vi "rs3 send_and_receive_raw_data3.vi"(0 "device in":u64=2630156989648, 2 "x1,y1,x2,y2":sgl[](array[numeric])=[0.0, 0.0, 0.0, 0.0], 5 "Send command":T3(ring)=enum."Distortion Centers", 7 "Input data":u32 format="%x", 9 "Input Intermediate Calibration Parameters":T2={"fx"=0.4987139, "fy"=0.7959354, "px"=0.49842373, "py"=0.49641025, "k left"=[-0.056493655, 0.06423295, 0.00075629074, -0.00050474313, -0.019832378], "fx2"=0.50020504, "fy2"=0.7982992, "py2"=0.5080532, "px2"=0.4993604, "k right"=[-0.056605, 0.065333016, 0.00090795365, 4.2479092e-05, -0.020946281], "RLeft"=[0.9999964, 0.001770121, -0.002005104, -0.0017697959, 0.9999984, 0.0001639397, 0.0020053908, -0.00016039048, 0.999998], "Rright"=[0.999991, -0.0020914313, -0.0036981972, 0.0020908315, 0.9999978, -0.00016603176, 0.0036985364, 0.00015829796, 0.99999315], "baseline"=-49.819336, "useBrownModel"=1, "1280x720"=[641.0225, 641.0225, 634.87134, 362.7353]}, 11 "error in (no error)":errorcluster, 13 "Calibration table input":T1={"version"=3, "table type"=60479, "table size"=496, "full version"=67109888, "crc32"=3963612841, "baseline"=-54.831806, "model"=1, "fx left"=917.7658, "fy left"=915.4345, "px left"=631.39185, "py left"=376.6227, "py right"=364.3492, "px right"=651.2822, "fy right"=921.49005, "fx right"=923.5849, "k left"=[0.13533829, -0.40519878, 0.0008784002, -0.0011180333, 0.3588802], "k right"=[0.12740475, -0.39763576, 0.00037952562, -0.0022863527, 0.35284942], "RLeft"=[0.9999986, 0.0009555143, -0.001359244, -0.0009574645, 0.9999985, -0.001434832, 0.001357871, 0.0014361315, 0.99999803], "Rright"=[0.99998456, -0.0019937593, -0.0051888847, 0.002001206, 0.99999696, 0.0014302958, 0.0051860176, -0.0014406577, 0.9999855], "uint8 reserved1"=[0, 0, 0, 0, 0, 0, 0, 0, 0, 0, 0, 0, 0, 0, 0, 0, 0, 0, 0, 0, 0, 0, 0, 0, 0, 0, 0, 0, 0, 0, 0, 0, 0, 0, 0, 0, 0, 0, 0, 0, 0, 0, 0, 0, 0, 0, 0, 0, 0, 0, 0, 0, 0, 0, 0, 0, 0, 0, 0, 0, 0, 0, 0, 0, 0, 0, 0, 0, 0, 0, 0, 0, 0, 0, 0, 0, 0, 0, 0, 0, 0, 0, 0, 0, 0, 0, 0, 0], "uint8 reserved2"=[0, 0, 0, 0, 0, 0, 0, 0, 0, 0, 0, 0, 0, 0, 0, 0, 0, 0, 0, 0, 0, 0, 0, 0, 0, 0, 0, 0, 0, 0, 0, 0, 0, 0, 0, 0, 0, 0, 0, 0, 0, 0, 0, 0, 0, 0, 0, 0, 0, 0, 0, 0, 0, 0, 0, 0, 0, 0, 0, 0, 0, 0, 0, 0], "1920x1080"=[1428.9095, 1428.9095, 951.85925, 556.0496], "1280x720"=[952.6064, 952.6064, 634.5728, 370.69974], "640x480"=[635.0709, 635.0709, 316.38187, 247.13316], "848x480"=[635.0709, 635.0709, 420.38187, 247.13316], "640x360"=[476.3032, 476.3032, 317.2864, 185.34987], "424x240"=[317.53546, 317.53546, 210.19093, 123.56658], "320x240"=[317.53546, 317.53546, 158.19093, 123.56658], "480x270"=[357.2274, 357.2274, 237.96481, 139.0124], "1280x800"=[1058.4515, 1058.4515, 633.9698, 411.8886], "960x540"=[714.4548, 714.4548, 475.92963, 278.0248], "Reserved1"=[714.4548, 714.4548, 475.92963, 278.0248], "Reserved 2"=[714.4548, 714.4548, 475.92963, 278.0248]} {"crc32" format="%x"}, 14 "Custom array":u8[](array[numeric])=[20, 1, 0, 0, 81, 0, 0, 0, 0, 0, 0, 0, 0, 0, 0, 0, 0, 0, 0, 0, 0, 0, 0, 0, 110, 87, 255, 62, 108, 194, 75, 63, 101, 49, 255, 62, 124, 41, 254, 62, 228, 101, 103, 189, 145, 140, 131, 61, 208, 65, 70, 58, 189, 80, 4, 186, 131, 119, 162, 188, 112, 13, 0, 63, 86, 93, 76, 63, 43, 172, 255, 62, 198, 15, 2, 63, 165, 218, 103, 189, 81, 205, 133, 61, 189, 3, 110, 58, 148, 43, 50, 56, 137, 151, 171, 188, 196, 255, 127, 63, 104, 3, 232, 58, 16, 104, 3, 187, 127, 248, 231, 186, 229, 255, 127, 63, 58, 231, 43, 57, 224, 108, 3, 59, 126, 46, 40, 185, 222, 255, 127, 63, 105, 255, 127, 63, 101, 16, 9, 187, 116, 93, 114, 187, 85, 6, 9, 59, 219, 255, 127, 63, 208, 24, 46, 185, 37, 99, 114, 59, 201, 252, 37, 57, 141, 255, 127, 63, 0, 71, 71, 194, 1, 0, 0, 0, 0, 0, 0, 0, 0, 0, 0, 0, 0, 0, 0, 0, 0, 0, 0, 0, 0, 0, 0, 0, 0, 0, 0, 0, 0, 0, 0, 0, 0, 0, 0, 0, 0, 0, 0, 0, 0, 0, 0, 0, 0, 0, 0, 0, 0, 0, 0, 0, 0, 0, 0, 0, 0, 0, 0, 0, 0, 0, 0, 0, 0, 0, 0, 0, 0, 0, 0, 0, 0, 0, 0, 0, 0, 0, 0, 0, 0, 0, 0, 0, 0, 0, 0, 0, 0, 0, 0, 0, 113, 65, 32, 68, 113, 65, 32, 68, 196, 183, 30, 68, 30, 94, 181, 67] format="%x") -> (1 "size(s)":i32=280, 3 "Output Calibration table":T1={"version"=3, "table type"=60479, "table size"=496, "full version"=67109888, "crc32"=3963612841, "baseline"=-54.831806, "model"=1, "fx left"=917.7658, "fy left"=915.4345, "px left"=631.39185, "py left"=376.6227, "py right"=364.3492, "px right"=651.2822, "fy right"=921.49005, "fx right"=923.5849, "k left"=[0.13533829, -0.40519878, 0.0008784002, -0.0011180333, 0.3588802], "k right"=[0.12740475, -0.39763576, 0.00037952562, -0.0022863527, 0.35284942], "RLeft"=[0.9999986, 0.0009555143, -0.001359244, -0.0009574645, 0.9999985, -0.001434832, 0.001357871, 0.0014361315, 0.99999803], "Rright"=[0.99998456, -0.0019937593, -0.0051888847, 0.002001206, 0.99999696, 0.0014302958, 0.0051860176, -0.0014406577, 0.9999855], "uint8 reserved1"=[0, 0, 0, 0, 0, 0, 0, 0, 0, 0, 0, 0, 0, 0, 0, 0, 0, 0, 0, 0, 0, 0, 0, 0, 0, 0, 0, 0, 0, 0, 0, 0, 0, 0, 0, 0, 0, 0, 0, 0, 0, 0, 0, 0, 0, 0, 0, 0, 0, 0, 0, 0, 0, 0, 0, 0, 0, 0, 0, 0, 0, 0, 0, 0, 0, 0, 0, 0, 0, 0, 0, 0, 0, 0, 0, 0, 0, 0, 0, 0, 0, 0, 0, 0, 0, 0, 0, 0], "uint8 reserved2"=[0, 0, 0, 0, 0, 0, 0, 0, 0, 0, 0, 0, 0, 0, 0, 0, 0, 0, 0, 0, 0, 0, 0, 0, 0, 0, 0, 0, 0, 0, 0, 0, 0, 0, 0, 0, 0, 0, 0, 0, 0, 0, 0, 0, 0, 0, 0, 0, 0, 0, 0, 0, 0, 0, 0, 0, 0, 0, 0, 0, 0, 0, 0, 0], "1920x1080"=[1428.9095, 1428.9095, 951.85925, 556.0496], "1280x720"=[952.6064, 952.6064, 634.5728, 370.69974], "640x480"=[635.0709, 635.0709, 316.38187, 247.13316], "848x480"=[635.0709, 635.0709, 420.38187, 247.13316], "640x360"=[476.3032, 476.3032, 317.2864, 185.34987], "424x240"=[317.53546, 317.53546, 210.19093, 123.56658], "320x240"=[317.53546, 317.53546, 158.19093, 123.56658], "480x270"=[357.2274, 357.2274, 237.96481, 139.0124], "1280x800"=[1058.4515, 1058.4515, 633.9698, 411.8886], "960x540"=[714.4548, 714.4548, 475.92963, 278.0248], "Reserved1"=[714.4548, 714.4548, 475.92963, 278.0248], "Reserved 2"=[714.4548, 714.4548, 475.92963, 278.0248]} {"crc32" format="%x"}, 4 "Sent Command":u8[](array[numeric])=[20, 0, 171, 205, 21, 0, 0, 0, 25, 0, 0, 0, 0, 0, 0, 0, 0, 0, 0, 0, 0, 0, 0, 0] format="%x", 6 "Response array":u8[](array[numeric])=[255, 255, 255, 255, 0, 0, 0, 0] format="%x", 8 "device out":u64=2630156989648, 10 "error":u64, 12 "Output Intermediate Calibration":T2, 15 "error out":errorcluster)   [LabVIEW 2017, in "libRealSense3.lvlib"]
doc: "Sends and receives raw data directly to device"
uses:
  libRealSense3.lvlib
  realsense2.dll
panel:
  out "Bad command":u8[](array[numeric])
  out "size(s) 2":i32
  out "TestCal":u8[](array[numeric])
  out "size out":i32
  out "size":i32=508
  out "new size?":u32
  # "RS3 Send & Receive"
  # "1B= 0001 1011\n23= 0010 0011\n21= 0010 0001"
  # "(C) 2017 Intel Corp.,  AGJ"
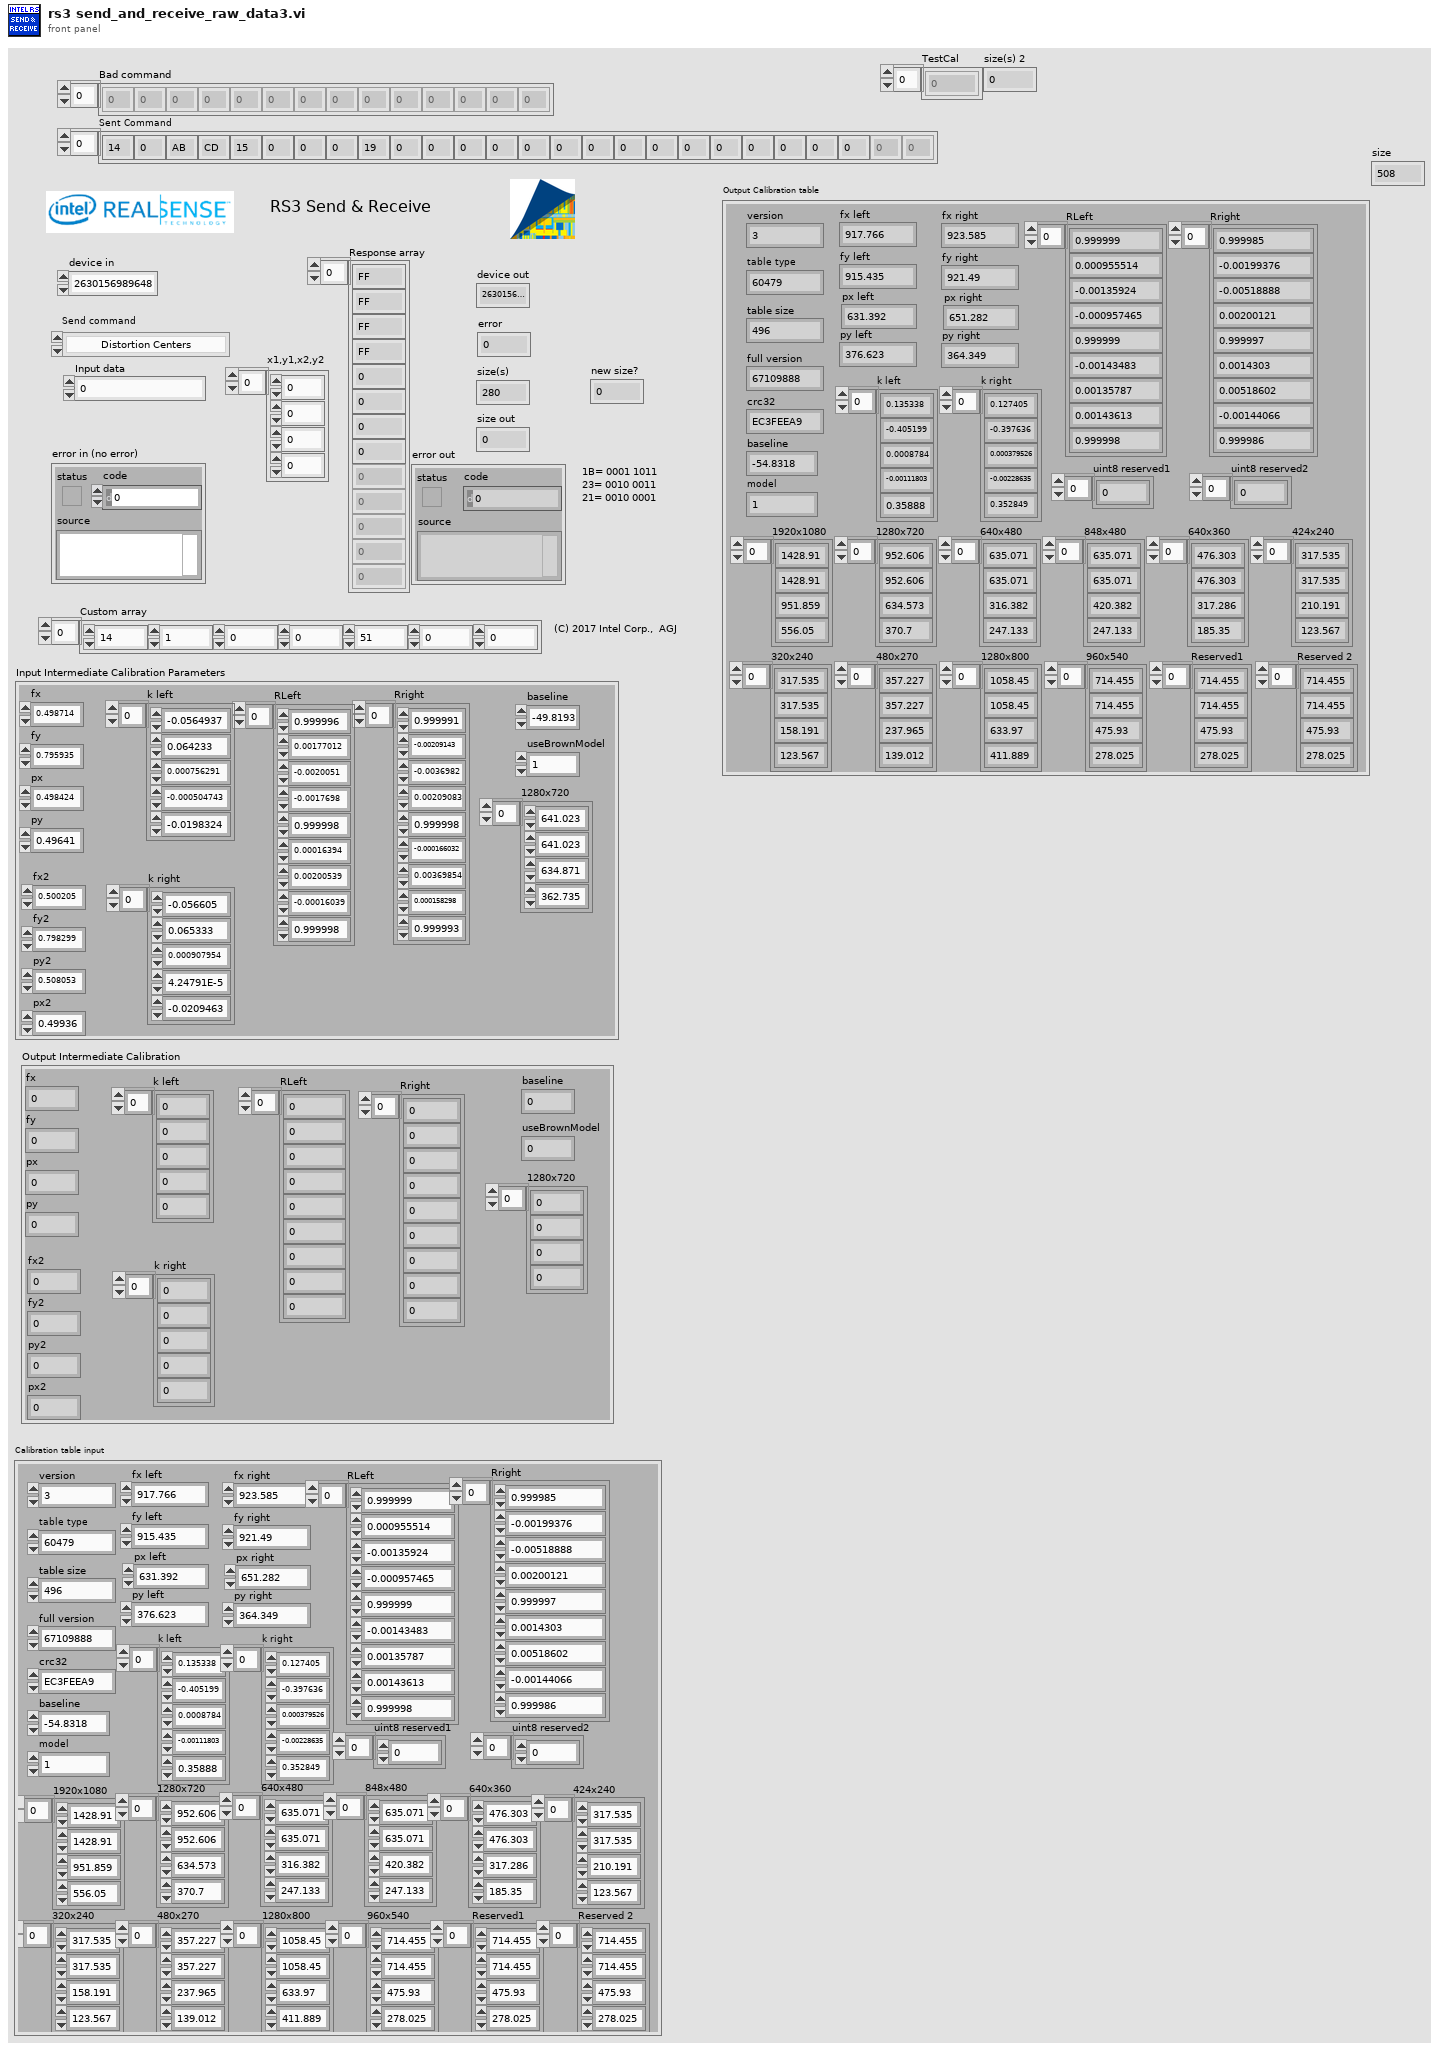
[diagram p1: front panel]
types:
  T1 = cluster{"version":u16, "table type":u16, "table size":u32, "full version":u32, "crc32":u32, "baseline":sgl, "model":u32, "fx left":sgl, "fy left":sgl, "px left":sgl, "py left":sgl, "py right":sgl, "px right":sgl, "fy right":sgl, "fx right":sgl, "k left":sgl[], "k right":sgl[], "RLeft":sgl[], "Rright":sgl[], "uint8 reserved1":u8[], "uint8 reserved2":u8[], "1920x1080":sgl[], "1280x720":sgl[], "640x480":sgl[], "848x480":sgl[], "640x360":sgl[], "424x240":sgl[], "320x240":sgl[], "480x270":sgl[], "1280x800":sgl[], "960x540":sgl[], "Reserved1":sgl[], "Reserved 2":sgl[]}
  T2 = cluster{"fx":sgl, "fy":sgl, "px":sgl, "py":sgl, "k left":sgl[], "fx2":sgl, "fy2":sgl, "py2":sgl, "px2":sgl, "k right":sgl[], "RLeft":sgl[], "Rright":sgl[], "baseline":sgl, "useBrownModel":u32, "1280x720":sgl[]}
  T3 = enum16{"GetCoefficientsData", "SetCoefficientsData", "SetIntermediateCoeffData", "GetDepthCalibData", "SetDepthCalibData", "GetRGBCalibData", "SetRGBCalibData", "RestoreFactoryCalib", "Read FSIN enable", "Turn on FSIN", "Turn off FSIN", "CAM master", "CAM slave", "CAM default", "Reset Header timestamp", "Query Mono/Bayer", "Write Mono", "Write Bayer", "Read Left center", "C0B0 Left Center X", "Shadow Update", "Distortion Centers", "Custom"}
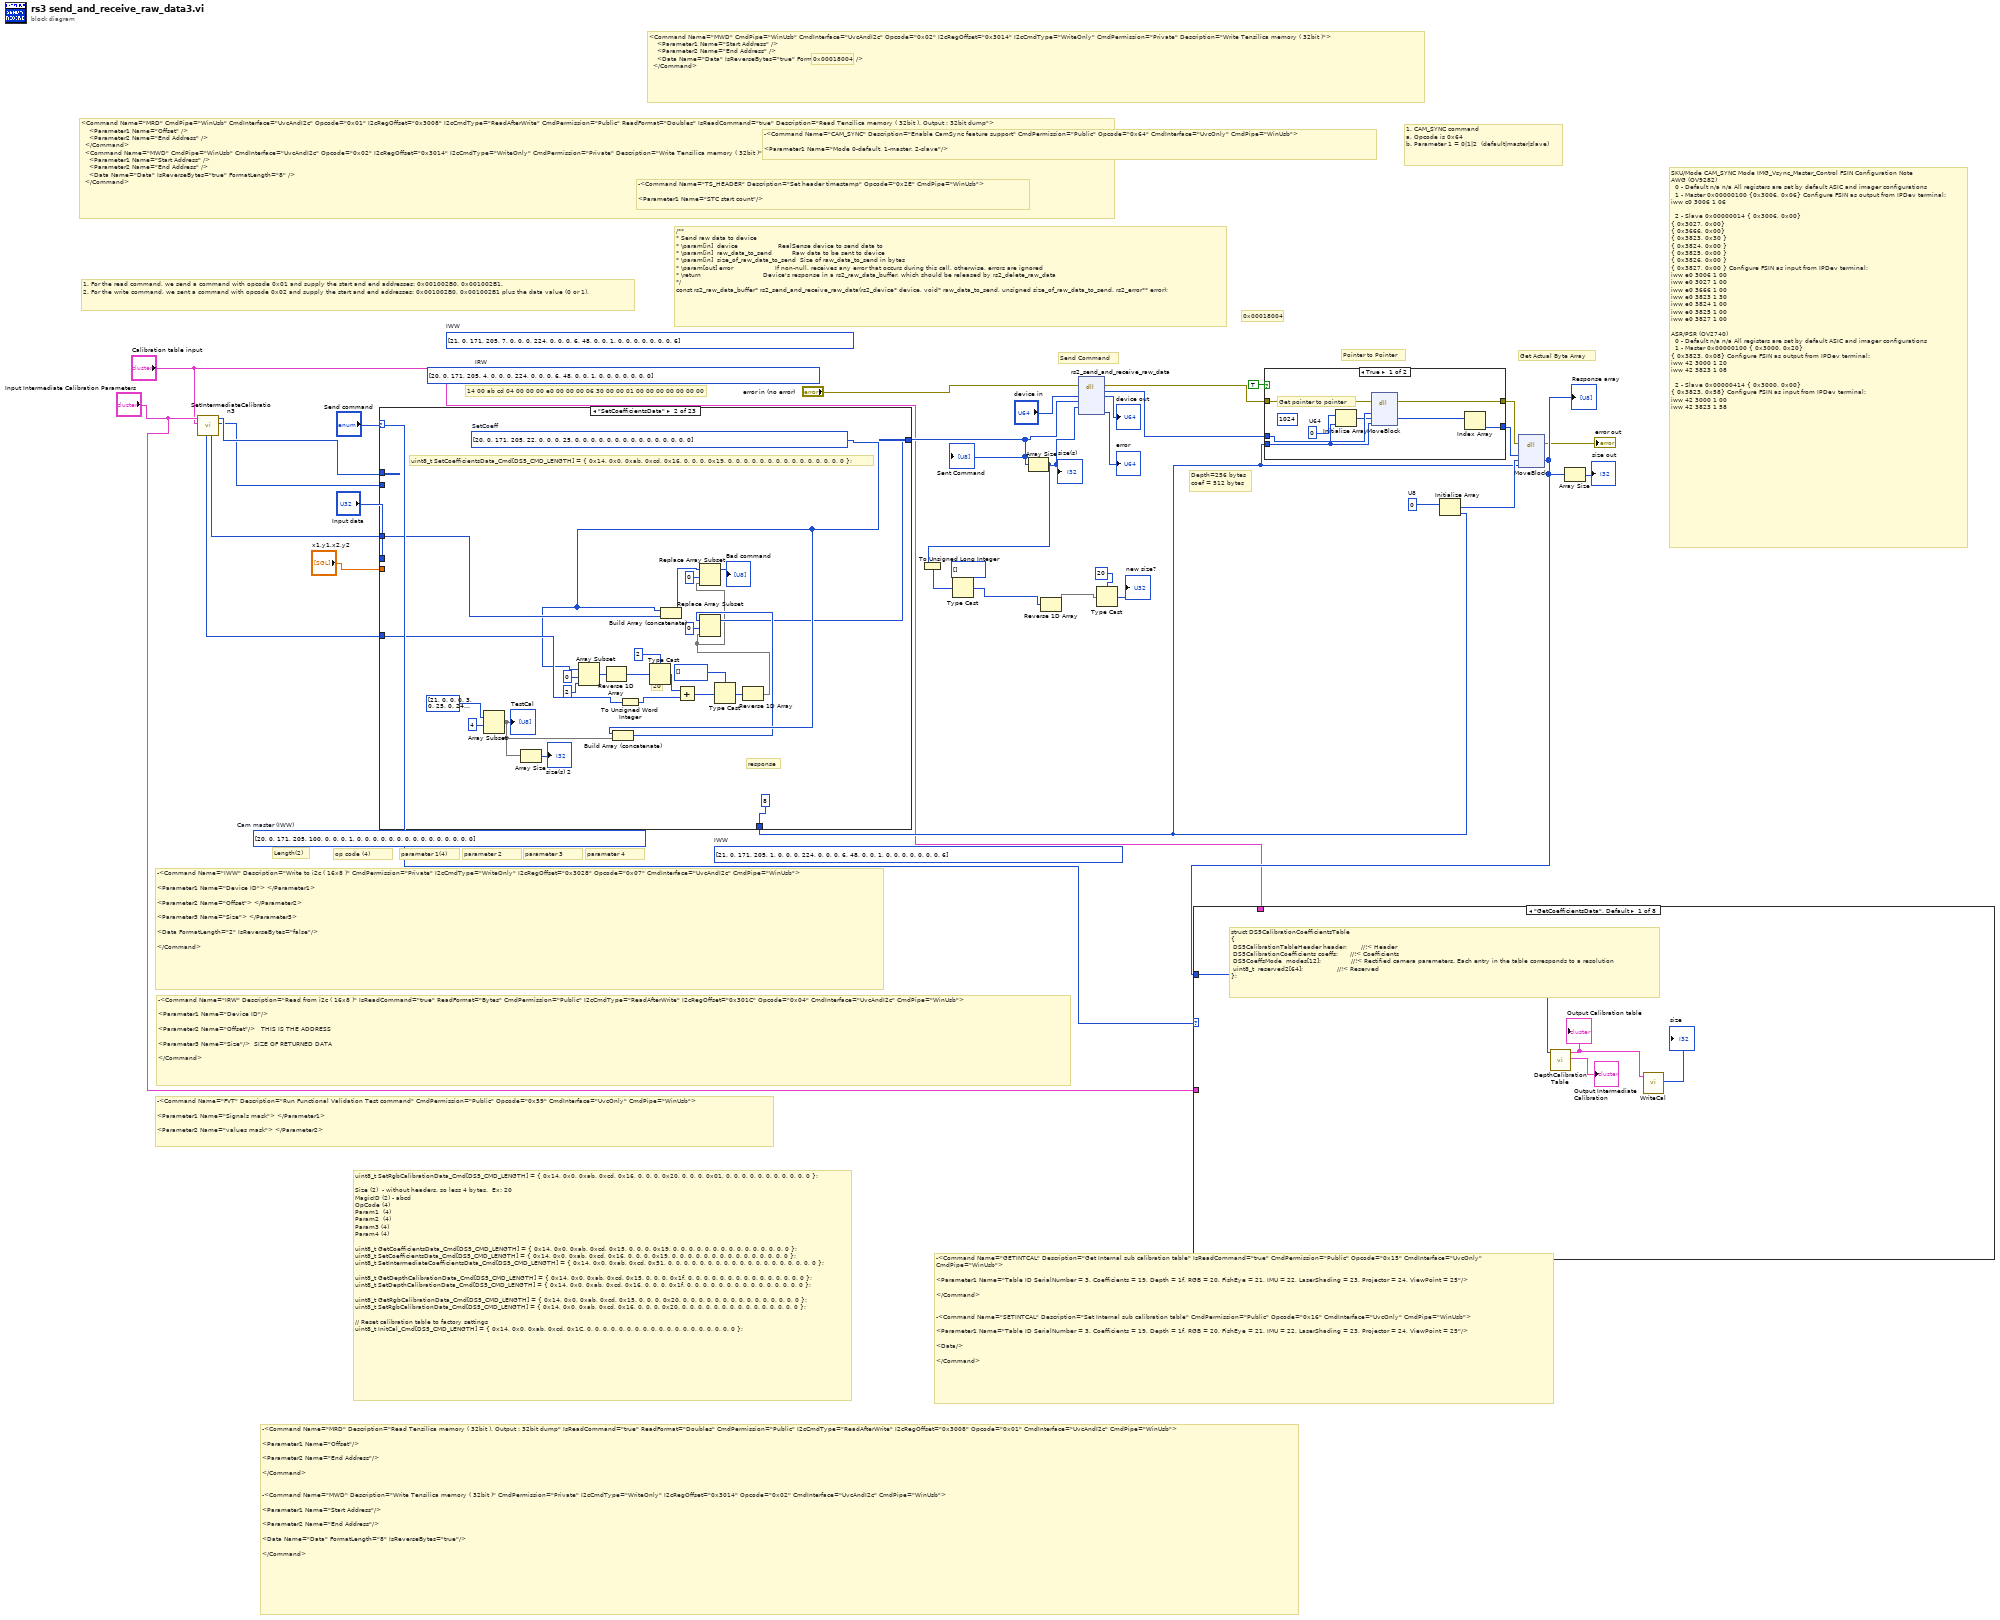
[diagram p0: block diagram]
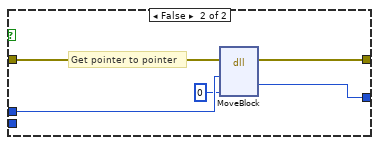
[diagram p2: hidden frame]
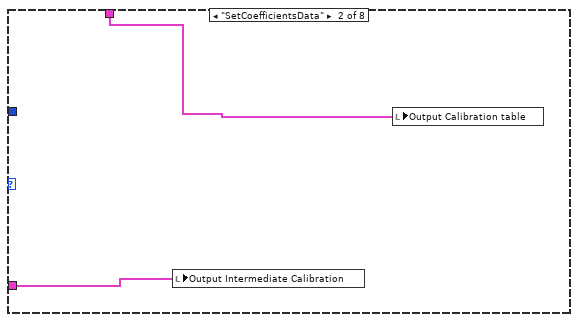
[diagram p3: hidden frame]
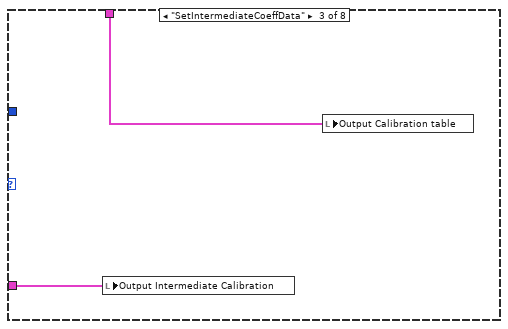
[diagram p4: hidden frame]
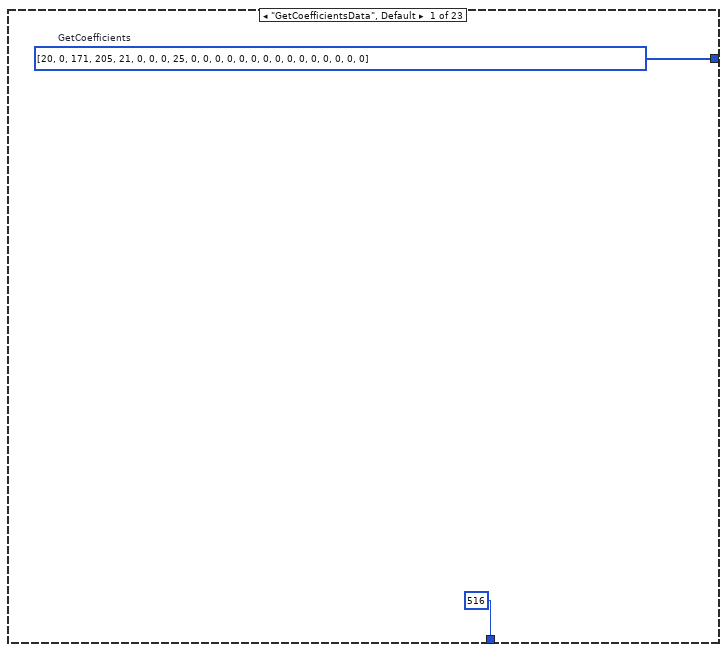
[diagram p10: hidden frame]
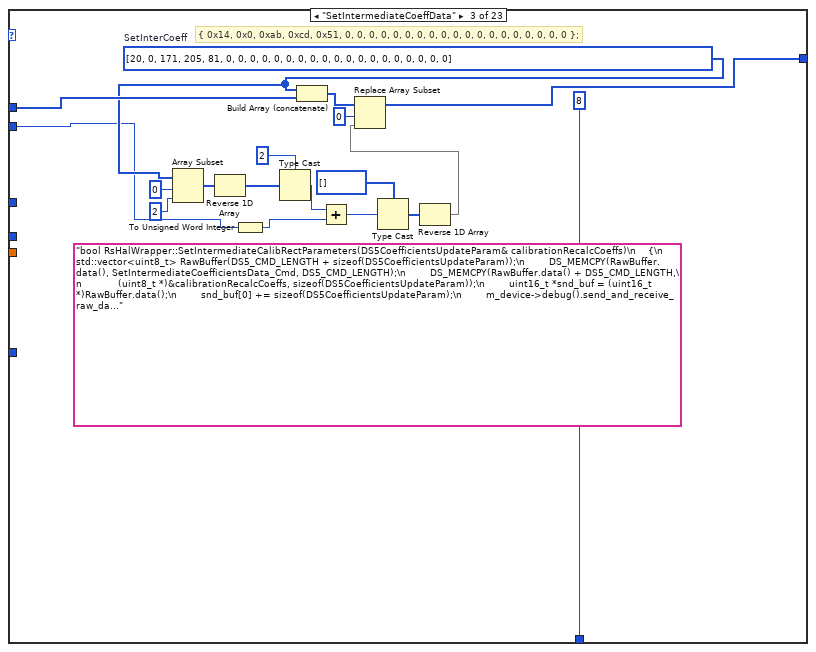
[diagram p11: hidden frame]
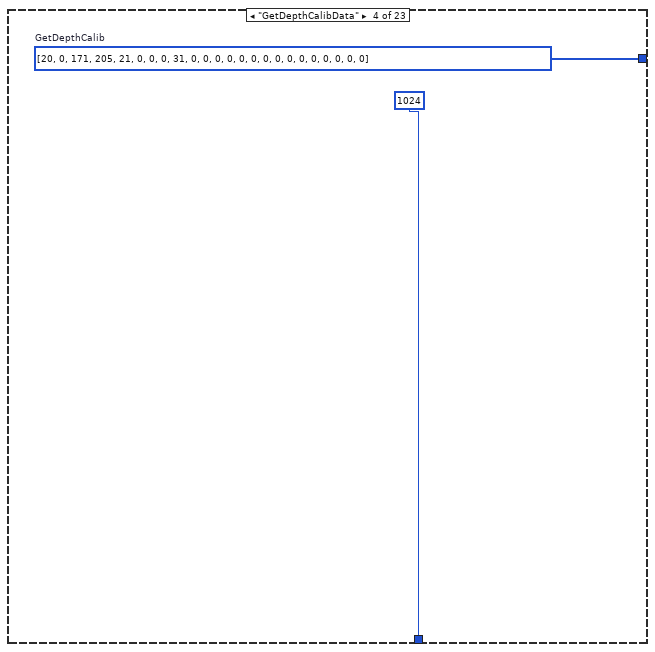
[diagram p12: hidden frame]
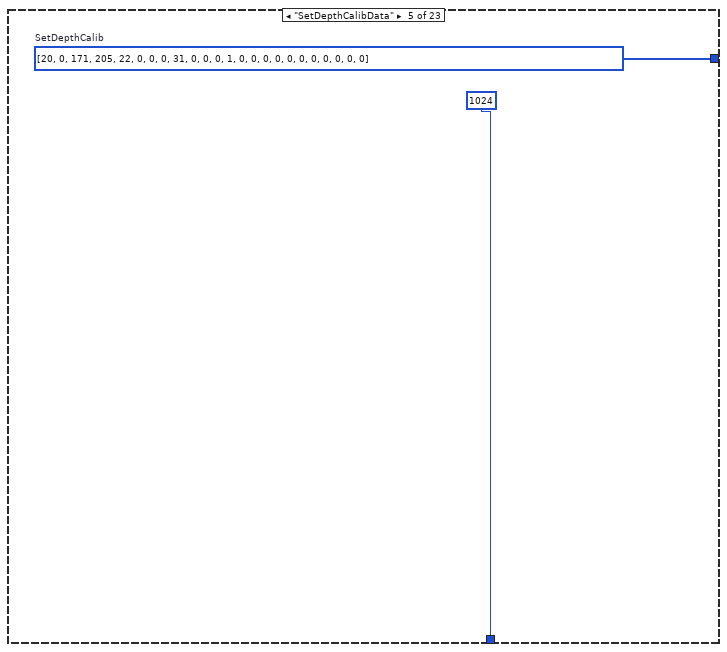
[diagram p13: hidden frame]
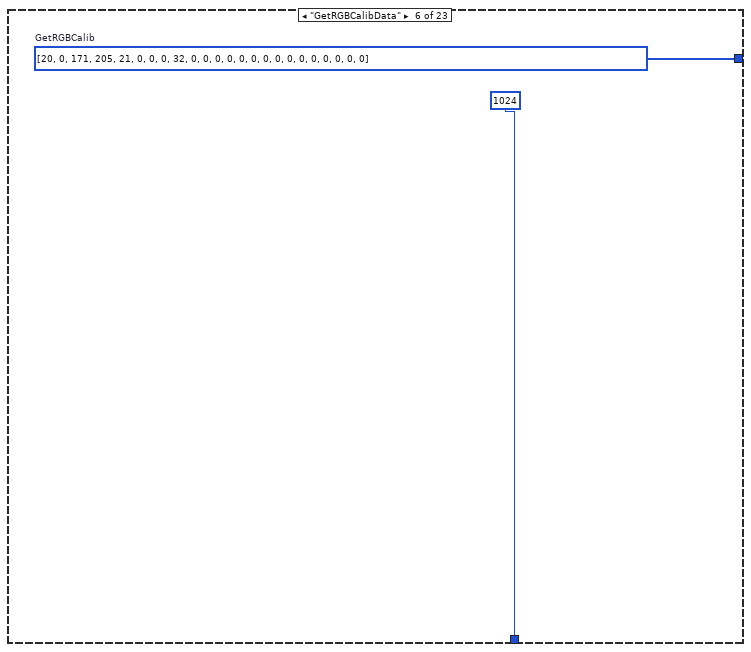
[diagram p14: hidden frame]
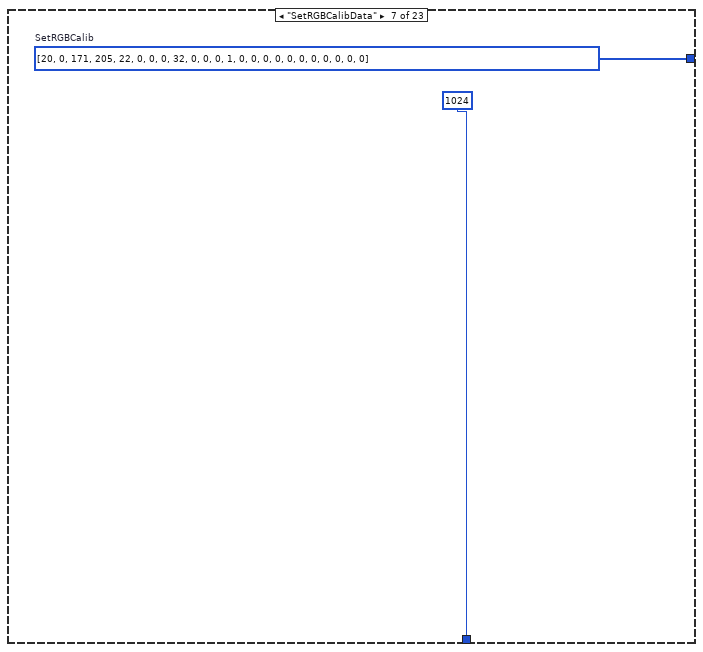
[diagram p15: hidden frame]
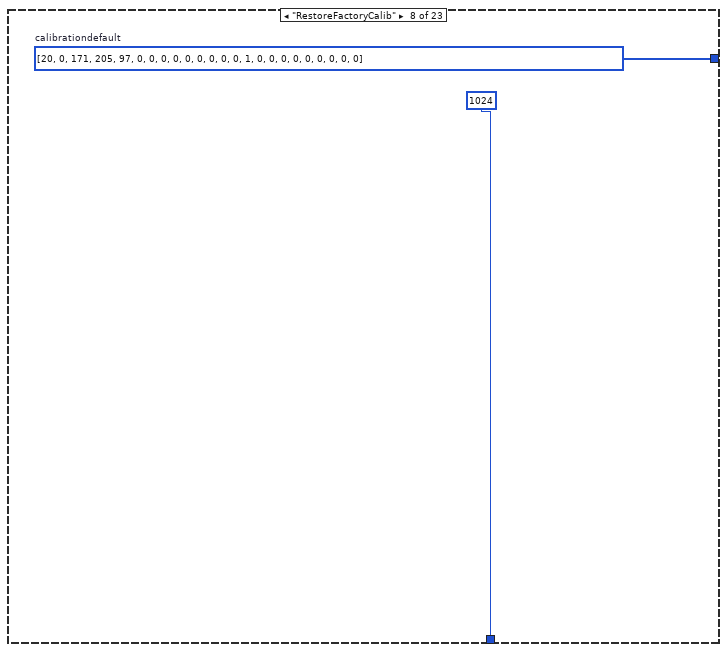
[diagram p16: hidden frame]
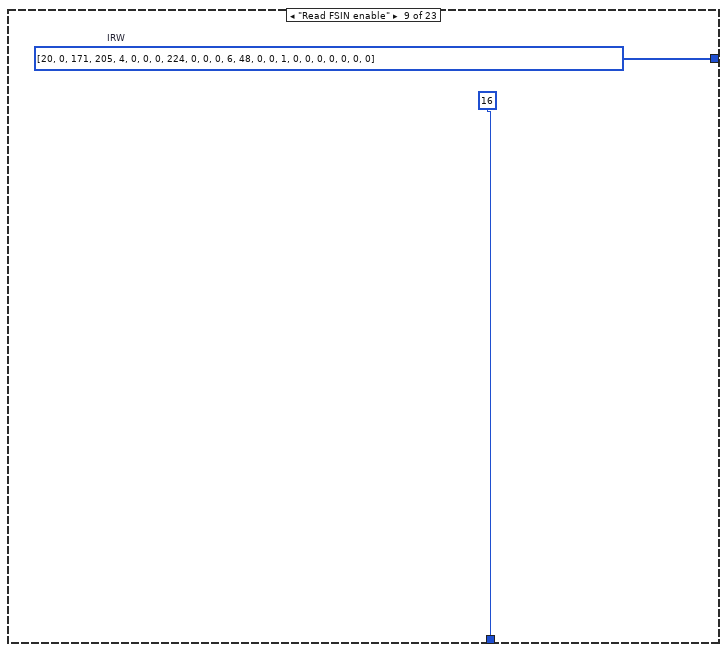
[diagram p17: hidden frame]
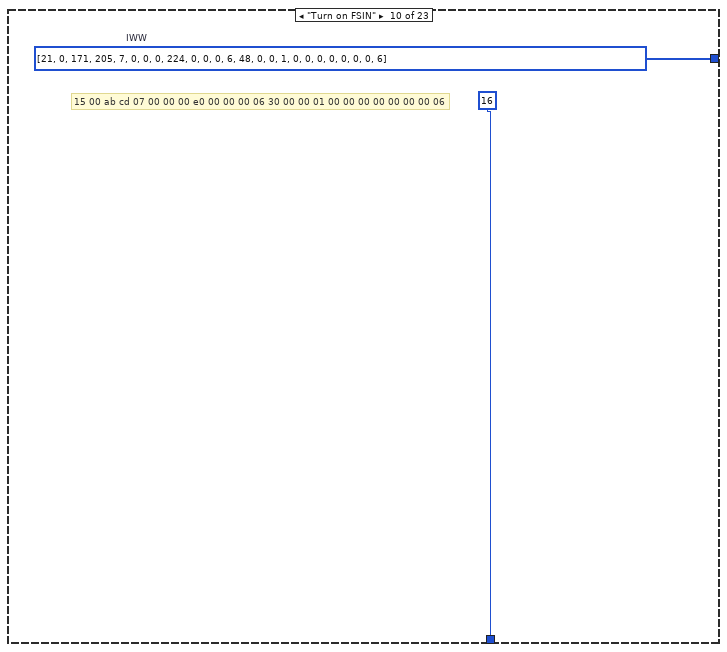
[diagram p18: hidden frame]
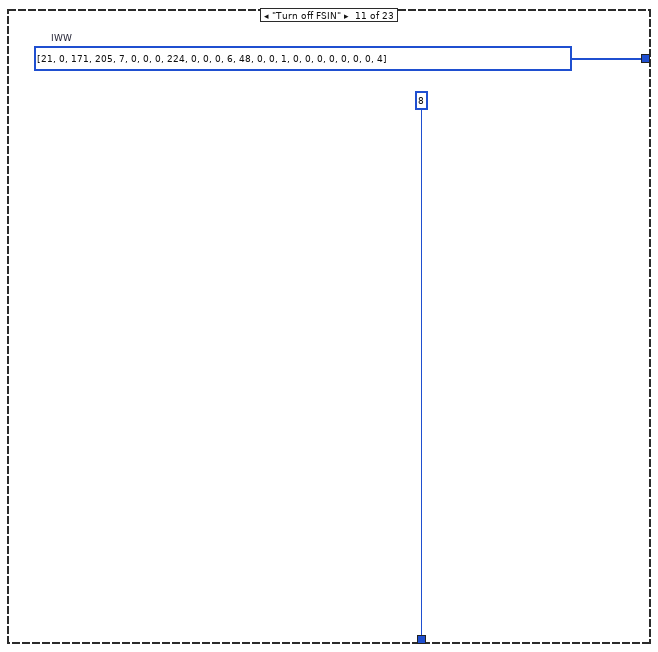
[diagram p19: hidden frame]
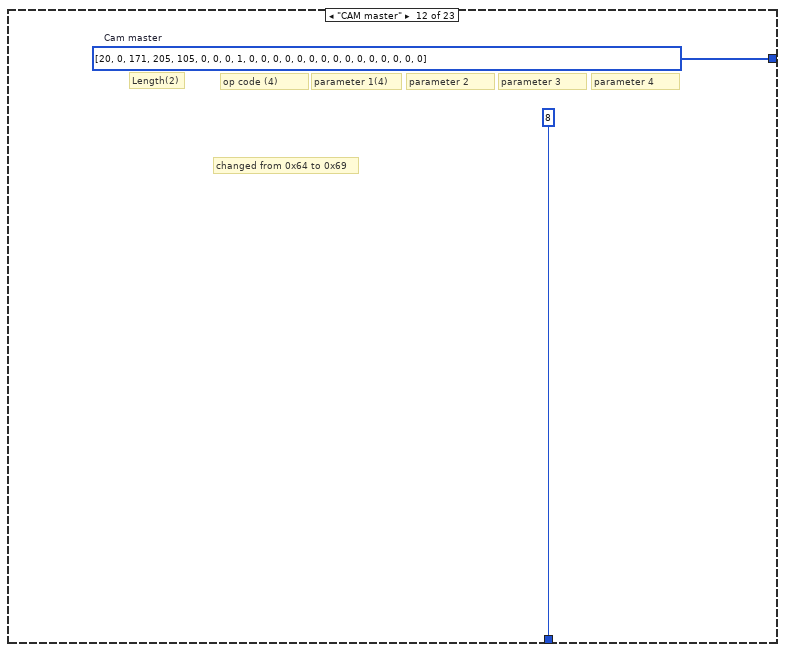
[diagram p20: hidden frame]
diagram:
  (unwired) u8[] [20, 0, 171, 205, 4, 0, 0, 0, 224, 0, 0, 0, 6, 48, 0, 0, 1, 0, 0, 0, 0, 0, 0, 0]  # IRW
  (unwired) u8[] [21, 0, 171, 205, 1, 0, 0, 0, 224, 0, 0, 0, 6, 48, 0, 0, 1, 0, 0, 0, 0, 0, 0, 0, 6]  # IWW
  (unwired) u8[] [20, 0, 171, 205, 100, 0, 0, 0, 1, 0, 0, 0, 0, 0, 0, 0, 0, 0, 0, 0, 0, 0, 0, 0]  # Cam master (IWW)
  (unwired) u8[] [21, 0, 171, 205, 7, 0, 0, 0, 224, 0, 0, 0, 6, 48, 0, 0, 1, 0, 0, 0, 0, 0, 0, 0, 6]  # IWW
  w26 = u8 0  # U8
  # "-<Command Name=\"MRD\" Description=\"Read Tensilica memory ( 32bit ). Output : 32bit dump\" IsReadCommand=\"true\" ReadFormat=\"Doubles\" CmdPermission=\"Public\" I2cCmdType=\"ReadAfterWrite\" I2cRegOffset=\"0x3008\" Opcode=\"0x01\" CmdInterface=\"UvcAndI2c\" CmdPipe=\"WinUsb\">\n\n<Parameter1 Name=\"Offset\"/>\n\n<Parameter2 Name=\"End Address\"/>\n\n</Command>\n\n\n-<Command Name=\"MWD\" Description=\"Write Tensilica memory ( 32bit )\" CmdPermission=\"Private\" I2cCmdType=\"WriteOnly\" I2cRegOffset=\"0x3014\" Opcode=\"0x02\" CmdInterface=\"UvcAndI2c\" CmdPipe=\"WinUsb\">\n\n<Parameter1 Name=\"Start Address\"/>\n\n<Parameter2 Name=\"End Address\"/>\n\n<Data Name=\"Data\" FormatLength=\"8\" IsReverseBytes=\"true\"/>\n\n</Command>"
  # "Get Actual Byte Array"
  # "Pointer to Pointer"
  # "<Command Name=\"MRD\" CmdPipe=\"WinUsb\" CmdInterface=\"UvcAndI2c\" Opcode=\"0x01\" I2cRegOffset=\"0x3008\" I2cCmdType=\"ReadAfterWrite\" CmdPermission=\"Public\" ReadFormat=\"Doubles\" IsReadCommand=\"true\" Description=\"Read Tensilica memory ( 32bit ). Output : 32bit dump\">\n    <Parameter1 Name=\"Offset\" />\n    <Parameter2 Name=\"End Address\" />\n  </Command>\n  <Command Name=\"MWD\" CmdPipe=\"WinUsb\" CmdInterface=\"UvcAndI2c\" Opcode=\"0x02\" I2cRegOffset=\"0x3014\" I2cCmdType=\"WriteOnly\" CmdPermission=\"Private\" Description=\"Write Tensilica memory ( 32bit )\">\n    <Parameter1 Name=\"Start Address\" />\n    <Parameter2 Name=\"End Address\" />\n    <Data Name=\"Data\" IsReverseBytes=\"true\" FormatLength=\"8\" />\n  </Command>"
  # "Length(2)"
  # "parameter 4"
  # "parameter 3"
  # "parameter 2"
  # "parameter 1(4)"
  # "op code (4)"
  # "1.\tFor the read command, we send a command with opcode 0x01 and supply the start and end addresses: 0x001002B0, 0x001002B1.\n2.\tFor the write command, we sent a command with opcode 0x02 and supply the start and end addresses: 0x001002B0, 0x001002B1 plus the data value (0 or 1)."
  # "0x00018004"
  # "0x00018004"
  # "<Command Name=\"MWD\" CmdPipe=\"WinUsb\" CmdInterface=\"UvcAndI2c\" Opcode=\"0x02\" I2cRegOffset=\"0x3014\" I2cCmdType=\"WriteOnly\" CmdPermission=\"Private\" Description=\"Write Tensilica memory ( 32bit )\">\n    <Parameter1 Name=\"Start Address\" />\n    <Parameter2 Name=\"End Address\" />\n    <Data Name=\"Data\" IsReverseBytes=\"true\" FormatLength=\"8\" />\n  </Command>"
  # "-<Command Name=\"CAM_SYNC\" Description=\"Enable CamSync feature support\" CmdPermission=\"Public\" Opcode=\"0x64\" CmdInterface=\"UvcOnly\" CmdPipe=\"WinUsb\">\n\n<Parameter1 Name=\"Mode 0-default, 1-master, 2-slave\"/>"
  # "SKU/Mode\tCAM_SYNC Mode\tIMG_Vsync_Master_Control\tFSIN Configuration\tNote\nAWG (OV9282)\t \t \t \t \n \t0 - Default\tn/a\tn/a\tAll registers are set by default ASIC and imager configurations\n \t1 - Master\t0x00000100\t{0x3006, 0x06}\tConfigure FSIN as output from IPDev terminal:\niww c0 3006 1 06\n \n \t2 - Slave\t0x00000014\t{ 0x3006, 0x00}\n{ 0x3027, 0x00}\n{ 0x3666, 0x00}\n{ 0x3823, 0x30 }\n{ 0x3824, 0x00 }\n{ 0x3825, 0x00 }\n{ 0x3826, 0x00 }\n{ 0x3827, 0x00 }\tConfigure FSIN as input from IPDev terminal:\niww e0 3006 1 00\niww e0 3027 1 00\niww e0 3666 1 00\niww e0 3823 1 30\niww e0 3824 1 00\niww e0 3825 1 00\niww e0 3827 1 00\n \nASR/PSR (OV2740)\t \t \t \t \n \t0 - Default\tn/a\tn/a\tAll registers are set by default ASIC and imager configurations\n \t1 - Master\t0x00000100\t{ 0x3000, 0x20}\n{ 0x3823, 0x08}\tConfigure FSIN as output from IPDev terminal:\niww 42 3000 1 20\niww 42 3823 1 08\n \n \t2 - Slave\t0x00000414\t{ 0x3000, 0x00}\n{ 0x3823, 0x58}\tConfigure FSIN as input from IPDev terminal:\niww 42 3000 1 00\niww 42 3823 1 58"
  # "-<Command Name=\"TS_HEADER\" Description=\"Set header timestamp\" Opcode=\"0x2E\" CmdPipe=\"WinUsb\">\n\n<Parameter1 Name=\"STC start count\"/>"
  # "1.\tCAM_SYNC command\na.\tOpcode is 0x64\nb.\tParameter 1 = 0|1|2  (default|master|slave)"
  # "-<Command Name=\"IRW\" Description=\"Read from i2c ( 16x8 )\" IsReadCommand=\"true\" ReadFormat=\"Bytes\" CmdPermission=\"Public\" I2cCmdType=\"ReadAfterWrite\" I2cRegOffset=\"0x301C\" Opcode=\"0x04\" CmdInterface=\"UvcAndI2c\" CmdPipe=\"WinUsb\">\n\n<Parameter1 Name=\"Device ID\"/>\n\n<Parameter2 Name=\"Offset\"/>   THIS IS THE ADDRESS\n\n<Parameter3 Name=\"Size\"/>  SIZE OF RETURNED DATA\n\n</Command>"
  # "-<Command Name=\"IWW\" Description=\"Write to i2c ( 16x8 )\" CmdPermission=\"Private\" I2cCmdType=\"WriteOnly\" I2cRegOffset=\"0x3028\" Opcode=\"0x07\" CmdInterface=\"UvcAndI2c\" CmdPipe=\"WinUsb\">\n\n<Parameter1 Name=\"Device ID\"> </Parameter1>\n\n<Parameter2 Name=\"Offset\"> </Parameter2>\n\n<Parameter3 Name=\"Size\"> </Parameter3>\n\n<Data FormatLength=\"2\" IsReverseBytes=\"false\"/>\n\n</Command>"
  # "14 00 ab cd 04 00 00 00 e0 00 00 00 06 30 00 00 01 00 00 00 00 00 00 00"
  # "uint8_t SetRgbCalibrationData_Cmd[DS5_CMD_LENGTH] = { 0x14, 0x0, 0xab, 0xcd, 0x16, 0, 0, 0, 0x20, 0, 0, 0, 0x01, 0, 0, 0, 0, 0, 0, 0, 0, 0, 0, 0 };\n\nSize (2)  - without headers, so less 4 bytes.  Ex: 20\nMagicID (2) - abcd\nOpCode (4)\nParam1  (4)\nParam2  (4)\nParam3 (4)\nParam4 (4)\n\nuint8_t GetCoefficientsData_Cmd[DS5_CMD_LENGTH] = { 0x14, 0x0, 0xab, 0xcd, 0x15, 0, 0, 0, 0x19, 0, 0, 0, 0, 0, 0, 0, 0, 0, 0, 0, 0, 0, 0, 0 };\nuint8_t SetCoefficientsData_Cmd[DS5_CMD_LENGTH] = { 0x14, 0x0, 0xab, 0xcd, 0x16, 0, 0, 0, 0x19, 0, 0, 0, 0, 0, 0, 0, 0, 0, 0, 0, 0, 0, 0, 0 };\nuint8_t SetIntermediateCoefficientsData_Cmd[DS5_CMD_LENGTH] = { 0x14, 0x0, 0xab, 0xcd, 0x51, 0, 0, 0, 0, 0, 0, 0, 0, 0, 0, 0, 0, 0, 0, 0, 0, 0, 0, 0 };\n\nuint8_t GetDepthCalibrationData_Cmd[DS5_CMD_LENGTH] = { 0x14, 0x0, 0xab, 0xcd, 0x15, 0, 0, 0, 0x1f, 0, 0, 0, 0, 0, 0, 0, 0, 0, 0, 0, 0, 0, 0, 0 };\nuint8_t SetDepthCalibrationData_Cmd[DS5_CMD_LENGTH] = { 0x14, 0x0, 0xab, 0xcd, 0x16, 0, 0, 0, 0x1f, 0, 0, 0, 0, 0, 0, 0, 0, 0, 0, 0, 0, 0, 0, 0 };\n\nuint8_t GetRgbCalibrationData_Cmd[DS5_CMD_LENGTH] = { 0x14, 0x0, 0xab, 0xcd, 0x15, 0, 0, 0, 0x20, 0, 0, 0, 0, 0, 0, 0, 0, 0, 0, 0, 0, 0, 0, 0 };\nuint8_t SetRgbCalibrationData_Cmd[DS5_CMD_LENGTH] = { 0x14, 0x0, 0xab, 0xcd, 0x16, 0, 0, 0, 0x20, 0, 0, 0, 0, 0, 0, 0, 0, 0, 0, 0, 0, 0, 0, 0 };\n\n// Reset calibration table to factory settings\nuint8_t InitCal_Cmd[DS5_CMD_LENGTH] = { 0x14, 0x0, 0xab, 0xcd, 0x1C, 0, 0, 0, 0, 0, 0, 0, 0, 0, 0, 0, 0, 0, 0, 0, 0, 0, 0, 0 };"
  # "Send Command"
  # "Depth=256 bytes\ncoef = 512 bytes"
  # "-<Command Name=\"FVT\" Description=\"Run Functional Validation Test command\" CmdPermission=\"Public\" Opcode=\"0x59\" CmdInterface=\"UvcOnly\" CmdPipe=\"WinUsb\">\n\n<Parameter1 Name=\"Signals mask\"> </Parameter1>\n\n<Parameter2 Name=\"values mask\"> </Parameter2>"
  # "-<Command Name=\"GETINTCAL\" Description=\"Get Internal sub calibration table\" IsReadCommand=\"true\" CmdPermission=\"Public\" Opcode=\"0x15\" CmdInterface=\"UvcOnly\" CmdPipe=\"WinUsb\">\n\n<Parameter1 Name=\"Table ID SerialNumber = 3, Coefficients = 19, Depth = 1f, RGB = 20, FishEye = 21, IMU = 22, LaserShading = 23, Projector = 24, ViewPoint = 25\"/>\n\n</Command>\n\n\n-<Command Name=\"SETINTCAL\" Description=\"Set Internal sub calibration table\" CmdPermission=\"Public\" Opcode=\"0x16\" CmdInterface=\"UvcOnly\" CmdPipe=\"WinUsb\">\n\n<Parameter1 Name=\"Table ID SerialNumber = 3, Coefficients = 19, Depth = 1f, RGB = 20, FishEye = 21, IMU = 22, LaserShading = 23, Projector = 24, ViewPoint = 25\"/>\n\n<Data/>\n\n</Command>"
  # "/**\n* Send raw data to device\n* \\param[in]  device                    RealSense device to send data to\n* \\param[in]  raw_data_to_send          Raw data to be sent to device\n* \\param[in]  size_of_raw_data_to_send  Size of raw_data_to_send in bytes\n* \\param[out] error                     If non-null, receives any error that occurs during this call, otherwise, errors are ignored\n* \\return                               Device's response in a rs2_raw_data_buffer, which should be released by rs2_delete_raw_data\n*/\nconst rs2_raw_data_buffer* rs2_send_and_receive_raw_data(rs2_device* device, void* raw_data_to_send, unsigned size_of_raw_data_to_send, rs2_error** error);"
  n1 = call "SetIntermediateCalibration3.vi"("Calibration table"="Calibration table input", "Input Calibration Parameters"="Input Intermediate Calibration Parameters") -> ("size(s)"=w17:i32, "Intermediate Output"=w18:u8[], "New Full cal. output"=w5:u8[], "New size full"=w4:i32)  [unwired: 4 in, 2 out]
  n2 = case shown="\"SetCoefficientsData\"" "Send command" {
    tunnel: [w34 w39 w73 w79 w81 w83 w85 w87 w89 w91 w93 w95 w97 w99 w100 w102 w104 w125 w128 w130 w132 w134 "Custom array"] -> w16
    tunnel: [516 ("Size") 8 ("Size") 8 ("Size") 1024 ("Size") 1024 ("Size") 1024 ("Size") 1024 ("Size") 1024 ("Size") 16 ("Size") 16 ("Size") 8 ("Size") 8 ("Size") 8 ("Size") 8 ("Size") 8 ("Size") 8 ("Size") 8 ("Size") 8 ("Size") 8 ("Size") 8 ("Size") 8 ("Size") 8 ("Size") 8 ("Size")] -> w19
    tunnel: w18 -> [_ _ w76 _ _ _ _ _ _ _ _ _ _ _ _ _ _ _ _ _ _ _ _]
    tunnel: w17 -> [_ _ w61 _ _ _ _ _ _ _ _ _ _ _ _ _ _ _ _ _ _ _ _]
    tunnel: "Input data" -> [_ _ _ _ _ _ _ _ _ _ _ _ _ _ _ _ w108 _ _ _ _ _ _]
    tunnel: "x1,y1,x2,y2" -> [_ _ _ _ _ _ _ _ _ _ _ _ _ _ _ _ _ w124 _ _ _ _ _]
    tunnel: w5 -> [_ w47 _ _ _ _ _ _ _ _ _ _ _ _ _ _ _ _ _ _ _ _ _]
    tunnel: w4 -> [_ w46 _ _ _ _ _ _ _ _ _ _ _ _ _ _ _ _ _ _ _ _ _]
    frame "GetCoefficientsData", Default {
      w34 = u8[] [20, 0, 171, 205, 21, 0, 0, 0, 25, 0, 0, 0, 0, 0, 0, 0, 0, 0, 0, 0, 0, 0, 0, 0]  # GetCoefficients
    }
    frame "SetCoefficientsData" {
      w42 = u8[] [20, 0, 171, 205, 22, 0, 0, 0, 25, 0, 0, 0, 0, 0, 0, 0, 0, 0, 0, 0, 0, 0, 0, 0]  # SetCoeff
      # "20"
      # "response"
      # "uint8_t SetCoefficientsData_Cmd[DS5_CMD_LENGTH] = { 0x14, 0x0, 0xab, 0xcd, 0x16, 0, 0, 0, 0x19, 0, 0, 0, 0, 0, 0, 0, 0, 0, 0, 0, 0, 0, 0, 0 };"
      n3 = Array Subset(array=u8[] [21, 0, 0, 0, 3, 0, 25, 0, 240, 1, 0, 0, 1, 4, 0, 4, 197, 74, 164, 177, 100, 161, 53, 63, 167, 130, 161, 63, 9, 183, 252, 62, 34, 237, 245, 62, 173, 102, 13, 62, 97, 181, 210, 190, 223, 192, 225, 57, 64, 135, 246, 57, 240, 121, 178, 62, 169, 97, 54, 63, 113, 40, 162, 63, 63, 247, 254, 62, 179, 217, 239, 62, 178, 73, 16, 62, 133, 99, 218, 190, 222, 124, 178, 185, 154, 53, 18, 58, 214, 202, 186, 62, 59, 255, 127, 63, 21, 159, 157, 187, 229, 200, 35, 58, 193, 119, 157, 59, 127, 253, 127, 63, 222, 52, 239, 59, 204, 251, 44, 186, 246, 26, 239, 187, 62, 254, 127, 63, 85, 255, 127, 63, 85, 110, 64, 57, 36, 189, 147, 187, 57, 238, 98, 185, 65, 254, 127, 63, 40, 36, 239, 187, 230, 176, 147, 59, 184, 43, 239, 59, 151, 253, 127, 63, 70, 157, 92, 194, 1, 0, 0, 0, 0, 0, 0, 0, 0, 0, 0, 0, 0, 0, 0, 0, 0, 0, 0, 0, 0, 0, 0, 0, 0, 0, 0, 0, 0, 0, 0, 0, 0, 0, 0, 0, 0, 0, 0, 0, 0, 0, 0, 0, 0, 0, 0, 0, 0, 0, 0, 0, 0, 0, 0, 0, 0, 0, 0, 0, 0, 0, 0, 0, 0, 0, 0, 0, 0, 0, 0, 0, 0, 0, 0, 0, 0, 0, 0, 0, 0, 0, 0, 0, 0, 0, 0, 0, 0, 0, 0, 0, 153, 66, 180, 68, 153, 66, 180, 68, 86, 90, 109, 68, 19, 71, 0, 68, 204, 88, 112, 68, 204, 88, 112, 68, 57, 60, 30, 68, 110, 9, 171, 67, 51, 59, 32, 68, 51, 59, 32, 68, 161, 165, 157, 67, 147, 12, 100, 67, 51, 59, 32, 68, 51, 59, 32, 68, 161, 165, 209, 67, 147, 12, 100, 67, 204, 88, 240, 67, 204, 88, 240, 67, 57, 60, 158, 67, 110, 9, 43, 67, 51, 59, 160, 67, 51, 59, 160, 67, 161, 165, 81, 67, 147, 12, 228, 66, 51, 59, 160, 67, 51, 59, 160, 67, 161, 165, 29, 67, 147, 12, 228, 66, 153, 66, 180, 67, 153, 66, 180, 67, 86, 90, 109, 67, 19, 71, 0, 67, 170, 134, 133, 68, 170, 134, 133, 68, 7, 10, 30, 68, 123, 10, 190, 67, 153, 66, 52, 68, 153, 66, 52, 68, 86, 90, 237, 67, 19, 71, 128, 67, 0, 0, 0, 0, 0, 0, 0, 0, 0, 0, 0, 0, 0, 0, 0, 0, 0, 0, 0, 0, 0, 0, 0, 0, 0, 0, 0, 0, 0, 0, 0, 0, 0, 0, 0, 0, 0, 0, 0, 0, 0, 0, 0, 0, 0, 0, 0, 0, 0, 0, 0, 0, 0, 0, 0, 0, 0, 0, 0, 0, 0, 0, 0, 0, 0, 0, 0, 0, 0, 0, 0, 0, 0, 0, 0, 0, 0, 0, 0, 0, 0, 0, 0, 0, 0, 0, 0, 0, 0, 0, 0, 0, 0, 0, 0, 0] ("Response array"), index=4) -> (w41:u8[])  [unwired: 1 in]
      "TestCal" <- w41
      n4 = Array Size(array=w41) -> (size(s)=→"size(s) 2":i32)
      n5 = Array Subset(array=w42, index=0, length=2) -> (w53:u8[])
      n6 = Reverse 1D Array(array=w53) -> (reversed array=w54:u8[])
      n7 = Build Array (concatenate)(w42, w41) -> (w40:u8[])
      n8 = To Unsigned Word Integer(number=w46) -> (unsigned 16bit integer=w48:u16)
      n9 = Type Cast(type=u16 2 ("length"), x=w54) -> (*(type *) &x=w55:u16)
      n10 = Build Array (concatenate)(w42, w47) -> (w37:u8[])
      n11 = Add(x=w55, y=w48) -> (x+y=w56:u16)
      n12 = Type Cast(type=u8[] [] ("subarray"), x=w56) -> (*(type *) &x=w57:u8[])
      n13 = Reverse 1D Array(array=w57) -> (reversed array=w36:u8[])
      n14 = Replace Array Subset(array=w37, new element=w36, index=0) -> (→"Bad command":u8[])
      n15 = Replace Array Subset(array=w40, new element=w36, index=0) -> (w39:u8[])
    }
    frame "SetIntermediateCoeffData" {
      (unwired) "bool RsHalWrapper::SetIntermediateCalibRectParameters(DS5CoefficientsUpdateParam& calibrationRecalcCoeffs)\n    {\n        std::vector<uint8_t> RawBuffer(DS5_CMD_LENGTH + sizeof(DS5CoefficientsUpdateParam));\n        DS_MEMCPY(RawBuffer.data(), SetIntermediateCoefficientsData_Cmd, DS5_CMD_LENGTH);\n        DS_MEMCPY(RawBuffer.data() + DS5_CMD_LENGTH,\n            (uint8_t *)&calibrationRecalcCoeffs, sizeof(DS5CoefficientsUpdateParam));\n        uint16_t *snd_buf = (uint16_t *)RawBuffer.data();\n        snd_buf[0] += sizeof(DS5CoefficientsUpdateParam);\n        m_device->debug().send_and_receive_raw_data(RawBuffer);\n\n        return true;\n    }"
      w63 = u8[] [20, 0, 171, 205, 81, 0, 0, 0, 0, 0, 0, 0, 0, 0, 0, 0, 0, 0, 0, 0, 0, 0, 0, 0]  # SetInterCoeff
      # "{ 0x14, 0x0, 0xab, 0xcd, 0x51, 0, 0, 0, 0, 0, 0, 0, 0, 0, 0, 0, 0, 0, 0, 0, 0, 0, 0, 0 };"
      n16 = Array Subset(array=w63, index=0, length=2) -> (w68:u8[])
      n17 = Reverse 1D Array(array=w68) -> (reversed array=w69:u8[])
      n18 = To Unsigned Word Integer(number=w61) -> (unsigned 16bit integer=w60:u16)
      n19 = Type Cast(type=u16 2 ("length"), x=w69) -> (*(type *) &x=w70:u16)
      n20 = Build Array (concatenate)(w63, w76) -> (w75:u8[])
      n21 = Add(x=w70, y=w60) -> (x+y=w71:u16)
      n22 = Type Cast(type=u8[] [] ("subarray"), x=w71) -> (*(type *) &x=w72:u8[])
      n23 = Reverse 1D Array(array=w72) -> (reversed array=w62:u8[])
      n24 = Replace Array Subset(array=w75, new element=w62, index=0) -> (w73:u8[])
    }
    frame "GetDepthCalibData" {
      w79 = u8[] [20, 0, 171, 205, 21, 0, 0, 0, 31, 0, 0, 0, 0, 0, 0, 0, 0, 0, 0, 0, 0, 0, 0, 0]  # GetDepthCalib
    }
    frame "SetDepthCalibData" {
      w81 = u8[] [20, 0, 171, 205, 22, 0, 0, 0, 31, 0, 0, 0, 1, 0, 0, 0, 0, 0, 0, 0, 0, 0, 0, 0]  # SetDepthCalib
    }
    frame "GetRGBCalibData" {
      w83 = u8[] [20, 0, 171, 205, 21, 0, 0, 0, 32, 0, 0, 0, 0, 0, 0, 0, 0, 0, 0, 0, 0, 0, 0, 0]  # GetRGBCalib
    }
    frame "SetRGBCalibData" {
      w85 = u8[] [20, 0, 171, 205, 22, 0, 0, 0, 32, 0, 0, 0, 1, 0, 0, 0, 0, 0, 0, 0, 0, 0, 0, 0]  # SetRGBCalib
    }
    frame "RestoreFactoryCalib" {
      w87 = u8[] [20, 0, 171, 205, 97, 0, 0, 0, 0, 0, 0, 0, 0, 0, 1, 0, 0, 0, 0, 0, 0, 0, 0, 0]  # calibrationdefault
    }
    frame "Read FSIN enable" {
      w89 = u8[] [20, 0, 171, 205, 4, 0, 0, 0, 224, 0, 0, 0, 6, 48, 0, 0, 1, 0, 0, 0, 0, 0, 0, 0]  # IRW
    }
    frame "Turn on FSIN" {
      w91 = u8[] [21, 0, 171, 205, 7, 0, 0, 0, 224, 0, 0, 0, 6, 48, 0, 0, 1, 0, 0, 0, 0, 0, 0, 0, 6]  # IWW
      # "15 00 ab cd 07 00 00 00 e0 00 00 00 06 30 00 00 01 00 00 00 00 00 00 00 06"
    }
    frame "Turn off FSIN" {
      w93 = u8[] [21, 0, 171, 205, 7, 0, 0, 0, 224, 0, 0, 0, 6, 48, 0, 0, 1, 0, 0, 0, 0, 0, 0, 0, 4]  # IWW
    }
    frame "CAM master" {
      w95 = u8[] [20, 0, 171, 205, 105, 0, 0, 0, 1, 0, 0, 0, 0, 0, 0, 0, 0, 0, 0, 0, 0, 0, 0, 0]  # Cam master
      # "changed from 0x64 to 0x69"
      # "Length(2)"
      # "parameter 4"
      # "parameter 3"
      # "parameter 2"
      # "parameter 1(4)"
      # "op code (4)"
    }
    frame "CAM slave" {
      w97 = u8[] [20, 0, 171, 205, 105, 0, 0, 0, 2, 0, 0, 0, 0, 0, 0, 0, 0, 0, 0, 0, 0, 0, 0, 0]  # Cam slave
      # "changed from 0x64 to 0x69"
      # "Length(2)"
      # "parameter 4"
      # "parameter 3"
      # "parameter 2"
      # "parameter 1(4)"
      # "op code (4)"
    }
    frame "CAM default" {
      w99 = u8[] [20, 0, 171, 205, 105, 0, 0, 0, 0, 0, 0, 0, 0, 0, 0, 0, 0, 0, 0, 0, 0, 0, 0, 0]  # Cam default
      # "changed from 0x64 to 0x69"
    }
    frame "Reset Header timestamp" {
      w100 = u8[] [20, 0, 171, 205, 46, 0, 0, 0, 0, 0, 0, 0, 0, 0, 0, 0, 0, 0, 0, 0, 0, 0, 0, 0]  # Set Header timestamp
    }
    frame "Query Mono/Bayer" {
      w102 = u8[] [20, 0, 171, 205, 1, 0, 0, 0, 176, 2, 16, 0, 180, 2, 16, 0, 0, 0, 0, 0, 0, 0, 0, 0]  # MRD
      # "Flip second bit to 0 for mono"
      # "0x001002B1"
      # "0x001002B0"
      # "Length(2)"
      # "parameter 4"
      # "parameter 3"
      # "parameter 2"
      # "parameter 1(4)"
      # "op code (4)"
    }
    frame "C0B0 Left Center X" {
      w106 = u8[] [24, 0, 171, 205, 2, 0, 0, 0, 96, 0, 16, 0, 100, 0, 16, 0, 0, 0, 0, 0, 0, 0, 0, 0]  # MWD
      # "data"
      # "0x00100064"
      # "0x00100060"
      # "end address"
      # "start address"
      # "Length(2)"
      # "parameter 4"
      # "parameter 3"
      # "parameter 2"
      # "parameter 1(4)"
      # "op code (4)"
      n25 = Type Cast(type=u8[] [0], x=w108) -> (*(type *) &x=w107:u8[])
      n26 = Reverse 1D Array(array=w107) -> (reversed array=w105:u8[])
      n27 = Build Array (concatenate)(w106, w105) -> (w104:u8[])
    }
    frame "Distortion Centers" {
      w119 = u8[] [0]
      w126 = u8[] [36, 0, 171, 205, 1, 3, 0, 0, 0, 0, 0, 0, 0, 0, 0, 0, 0, 0, 0, 0, 0, 0, 0, 0]  # Distortion center
      # "0x301"
      # "Length(2)"
      # "parameter 4"
      # "parameter 3"
      # "parameter 2"
      # "parameter 1(4)"
      # "op code (4)"
      n28 = Index Array(array=w124) -> (element #1=w123:sgl, element #2=w122:sgl, element #3=w121:sgl, element #4=w120:sgl)  [unwired: 4 in]
      n29 = Type Cast(type=w119, x=w123) -> (*(type *) &x=w118:u8[])
      n30 = Type Cast(type=w119, x=w122) -> (*(type *) &x=w116:u8[])
      n31 = Type Cast(type=w119, x=w121) -> (*(type *) &x=w114:u8[])
      n32 = Type Cast(type=w119, x=w120) -> (*(type *) &x=w111:u8[])
      n33 = Reverse 1D Array(array=w118) -> (reversed array=w117:u8[])
      n34 = Reverse 1D Array(array=w116) -> (reversed array=w115:u8[])
      n35 = Reverse 1D Array(array=w114) -> (reversed array=w113:u8[])
      n36 = Reverse 1D Array(array=w111) -> (reversed array=w112:u8[])
      n37 = Build Array (concatenate)(w126, w117, w115, w113, w112) -> (w125:u8[])
    }
    frame "Read Left center" {
      w128 = u8[] [20, 0, 171, 205, 1, 0, 0, 0, 96, 0, 16, 0, 100, 0, 16, 0, 0, 0, 0, 0, 0, 0, 0, 0]  # MRD
      # "Do I need to reverse?"
      # "data"
      # "0x00100064"
      # "0x00100060"
      # "end address"
      # "start address"
      # "Length(2)"
      # "parameter 4"
      # "parameter 3"
      # "parameter 2"
      # "parameter 1(4)"
      # "op code (4)"
    }
    frame "Shadow Update" {
      w130 = u8[] [20, 0, 171, 205, 17, 0, 0, 0, 255, 255, 255, 255, 0, 0, 0, 0, 0, 0, 0, 0, 0, 0, 0, 0]  # OTF Update(Shadow)
      # "FFFF\n0FF0"
      # "data"
      # "end address"
      # "start address"
      # "Length(2)"
      # "parameter 4"
      # "parameter 3"
      # "parameter 2"
      # "parameter 1(4)"
      # "op code (4)"
    }
    frame "Write Mono" {
      (unwired) u8[] [21, 0, 171, 205, 2, 0, 0, 0, 176, 2, 16, 0, 180, 2, 16, 0, 0, 0, 0, 0, 0, 0, 0, 0, 33]  # MWD
      w132 = u8[] [20, 0, 171, 205, 49, 0, 0, 0, 0, 0, 0, 0, 0, 0, 0, 0, 0, 0, 0, 0, 0, 0, 0, 0]  # MWD
      # "data"
      # "0x001002B4"
      # "0x001002B0"
      # "Length(2)"
      # "parameter 4"
      # "parameter 3"
      # "parameter 2"
      # "parameter 1(4)"
      # "op code (4)"
    }
    frame "Write Bayer" {
      (unwired) u8[] [21, 0, 171, 205, 2, 0, 0, 0, 176, 2, 16, 0, 180, 2, 16, 0, 0, 0, 0, 0, 0, 0, 0, 0, 35]  # MWD
      w134 = u8[] [20, 0, 171, 205, 49, 0, 0, 0, 1, 0, 0, 0, 0, 0, 0, 0, 0, 0, 0, 0, 0, 0, 0, 0]  # MWD
      # "Use opcode 0x31 and set param 1 to either 0 or 1.\n\nSETDEMOSAIC =         0x31, // SETDEMOSAIC, Write, Bytes, 1, \"Update demosaic mode\", \"0-demosaic off  1-demosaic on\""
      # "data"
      # "0x001002B4"
      # "0x001002B0"
      # "Length(2)"
      # "parameter 4"
      # "parameter 3"
      # "parameter 2"
      # "parameter 1(4)"
      # "op code (4)"
    }
    frame "Custom" {
    }
  }
  "Sent Command" <- w16
  n38 = Array Size(array=w16) -> (size(s)=w9:i32)
  "size(s)" <- w9
  n39 = To Unsigned Long Integer(number=w9) -> (unsigned 32bit integer=w11:u32)
  n40 = Type Cast(type=u8[] [] ("subarray"), x=w11) -> (*(type *) &x=w14:u8[])
  n41 = Reverse 1D Array(array=w14) -> (reversed array=w13:u8[])
  n42 = dll-call lib="C:/Users/agrunnet/Documents/libRealSense6/realsense2.dll" fn="rs2_send_and_receive_raw_data"(error in="error in (no error)", "device"="device in", "input buffer"=w16, "size"=w9) -> (error out=w28:errorcluster, "output buffer"=w27:u64, "device"=→"device out":u64, "error"=→"error":u64)  [unwired: 5 in, 1 out]
  n43 = Type Cast(type=u32 20 ("size(s)"), x=w13) -> (*(type *) &x=→"new size?":u32)
  n44 = case shown="True" TRUE {
    tunnel: w28 -> [w145 w150]
    tunnel: w27 -> [w144 w149]
    tunnel: [w140 w146] -> w8
    tunnel: [w139 w148] -> w22
    tunnel: w19 -> [w138 _]
    frame True {
      (unwired) 1024 ("dimension size")
      w142 = u64 0  # U64
      # "Get pointer to pointer"
      n45 = Initialize Array(w142, w138) -> (w143:u64[])
      n46 = dll-call lib="LabVIEW" fn="MoveBlock"(error in=w145, "Address(Pointer)"=w144, "Destination"=w143, "Size"=w138) -> (error out=w139:errorcluster, "Destination"=w141:u64[])  [unwired: 5 in, 1 out]
      n47 = Index Array(array=w141) -> (element=w140:u64)  [unwired: 1 in]
    }
    frame False {
      # "Get pointer to pointer"
      n48 = dll-call lib="LabVIEW" fn="MoveBlock"(error in=w150, "Address(Pointer)"=w149, "Size"=0) -> (error out=w148:errorcluster, "Destination"=w146:u64)  [unwired: 6 in, 1 out]
    }
  }
  n49 = Initialize Array(w26, w19) -> (w25:u8[])
  n50 = dll-call lib="LabVIEW" fn="MoveBlock"(error in=w22, "Address(Pointer)"=w8, "Destination"=w25, "Size"=w19) -> (error out=→"error out":errorcluster, "Destination"=w23:u8[])  [unwired: 5 in, 1 out]
  "Response array" <- w23
  n51 = case shown="\"GetCoefficientsData\", Default" "Send command" {
    tunnel: w23 -> [w151 _ _ _ _ _ _ _]
    tunnel: "Input Intermediate Calibration Parameters" -> [_ w155 w158 _ _ _ _ _]
    tunnel: "Calibration table input" -> [_ w156 w157 _ _ _ _ _]
    frame "GetCoefficientsData", Default {
      # "struct DS5CalibrationCoefficientsTable\n{\n\tDS5CalibrationTableHeader header;       //!< Header\n\tDS5CalibrationCoefficients coeffs;      //!< Coefficients\n\tDS5CoeffsMode  modes[12];               //!< Rectified camera parameters. Each entry in the table corresponds to a resolution\n\tuint8_t  reserved2[64];                 //!< Reserved\n};"
      n52 = call "DepthCalibrationTable.vi"("DS5CalibrationCoefficientsTable"=w151) -> ("New Calibration Parameters"=→"Output Intermediate Calibration":T2, "Calibration table"=w153:T1)  [unwired: 7 in, 2 out]
      "Output Calibration table" <- w153
      n53 = call "WriteCal.vi"("Calibration table"=w153) -> ("size"=→"size":i32)  [unwired: 9 in, 1 out]
    }
    frame "SetCoefficientsData" {
      n54 = local write "Output Intermediate Calibration"(w155) -> ()
      n55 = local write "Output Calibration table"(w156) -> ()
    }
    frame "SetIntermediateCoeffData" {
      n56 = local write "Output Intermediate Calibration"(w158) -> ()
      n57 = local write "Output Calibration table"(w157) -> ()
    }
    frame "GetDepthCalibData" {
      # "//! DS5 depth calibration table. Contains raw calibraiton data. Table ID = 0x1F.\nstruct DS5DepthCalibrationTable\n{\n\tDS5CalibrationTableHeader header;       //!< Header\n\tuint32_t rmax;                          //!< Maximum permissible rotation\n\tDS5CalIntrinsics instrinsicsLeft;       //!< Intrinsics of the left camera\n\tDS5CalIntrinsics instrinsicsRight;      //!< Intrinsics of the right camera\n\tfloat Kd[9];                            //!< Intrinsics of the depth camera at calibration resolution\n\tfloat Rd[3];                            //!< Rotation vector of the depth camera against world coordinates. Stored as Rodriguez rotation vector.\n\tfloat Td[3];                            //!< The new translation between non-rectified left and right camera, passed as T=-Rt, where t is the translation vector and R is the rotaion matrix\n\tuint16_t imageWidth;                    //!< Width of the images used during calibration\n\tuint16_t imageHeight;                   //!< Height of the images used during calibration\n\tuint16_t calibrationType;               //!< Calibration type\n\tuint8_t reserved[10];                   //!< Reserved\n};"
    }
    frame "SetDepthCalibData" {
    }
    frame "GetRGBCalibData" {
      # "struct DS5RGBCalibrationTable\n{\n\tDS5CalibrationTableHeader header;       //!< Header\n\tDS5CalIntrinsics intrinsics;            //!< Intrinsics of the RGB camera\n\tfloat P[12];                            //!< Projection matrix from depth to unrectified RGB camera\n\tuint16_t imageWidth;                    //!< Width of the images used during calibration\n\tuint16_t imageHeight;                   //!< Height of the images used during calibration\n\tfloat Krect[9];                         //!< Intrinsics of the rectified RGB camera\n\tfloat Rrect[9];                         //!< Inverse rotation of the RGB camera in rectified coordinate system\n\tfloat Trect[3];                         //!< Translation of the RGB camera in rectified coordinate system\n\tuint8_t reserved[24];                   //!< Reserved\n};"
    }
    frame "SetRGBCalibData" {
    }
    frame "RestoreFactoryCalib" {
    }
  }
  n58 = Array Size(array=w23) -> (size(s)=→"size out":i32)
